vi "chaim Tx poulse.vi"() -> ()   [LabVIEW 2021]
doc: "This template is for the Simple NI-USRP Streaming design, a design that shows the basics of streaming data to and from an NI USRP-294x/295x device. Refer to the block diagram for more information about how to use this template."
uses:
  <vilib>/userDefined/Silver/nirio_resource_slv.ctl
  Host/SubVIs/Start Trigger.ctl
  <vilib>/Utility/error.llb/Error Cluster From Error Code.vi
  <vilib>/rvi/errors/niLvFpgaAdjustHostInterfaceError.vi
  <vilib>/rvi/interface/nirviReadWriteControl/nirviReadWriteControl.xnode
  <vilib>/rvi/interface/nirviMethod/nirviMethod.xnode
  NiFpgaLv.dll
  <vilib>/rvi/interface/Simulation/niFpgaSimulationCallBeginRW.vi
  <vilib>/FPGAPlugInAG/Dynamic/niLvFpga_WriteFifo_Dynamic.vi
  <vilib>/rvi/errors/niLvFpgaMergeErrorWithErrorCode.vi
panel:
  out "error out":errorcluster
  in  "stop":bool
  out "polse gen 1 params":T1
  out "pulse read polse gen 1":u32
  out "tx ocupaied":bool[](array[boolean])
  out "poulse param":T1
  out "pulse read":u32
  out "fpga clock":u64
  out "reset system clock":bool
  out "data":u64[](array[numeric]) format="%#.4e"
  out "Empty Elements Remaining":u32
  in  "file path":path
  in  "config tab":enum32{"Tx Configuration"}(tab)
  in  "tx config":T3={"rf enable 0"=TRUE, "rf config 0"={"antenna"="TX1", "frequency"=2000000000.0, "lo frequency"=-1.0, "level"=0.0}, "rf enable 1"=TRUE, "rf config 1"={"antenna"="TX1", "frequency"=2000000000.0, "lo frequency"=-1.0, "level"=0.0}, "transfer mode"=enum."Finite", "sample rate"=10000000.0, "number of samples"=8192, "start trigger"=enum."Immediate", "tone frequency"=100000.0} {"tone frequency" format="%#.3pHz"; "sample rate" format="%#.3pS/s"; "rf config 0"."level" format="%#_gdBm"; "rf config 0"."lo frequency" format="%#.3pHz"; "rf config 0"."frequency" format="%#.3pHz"; "rf config 1"."level" format="%#_gdBm"; "rf config 1"."lo frequency" format="%#.3pHz"; "rf config 1"."frequency" format="%#.3pHz"}
  in  "USRP RIO device":T4="RIO0" caption="USRP RIO Device"
  in  "reference frequency source":string(combo)="Internal" caption="Reference Frequency Source"
  in  "indicator tab":T5(tab)
  out "tx.output waveform":waveform(dbl)[](graph) caption="Output Waveform"
  out "tx.coerced config":T6 caption="Tx" {"coerced sample rates" format="%#.3pS/s"; "coerced levels" format="%#.3gdBm"; "coerced lo frequencies" format="%#.3pHz"; "coerced frequencies" format="%#.3pHz"}
  # "This template is for the Simple NI-USRP Streaming design, a design that shows the basics of streaming data on a USRP RIO device. See the block diagram for more information on how to use this template."
  # "Simple Tx Streaming"
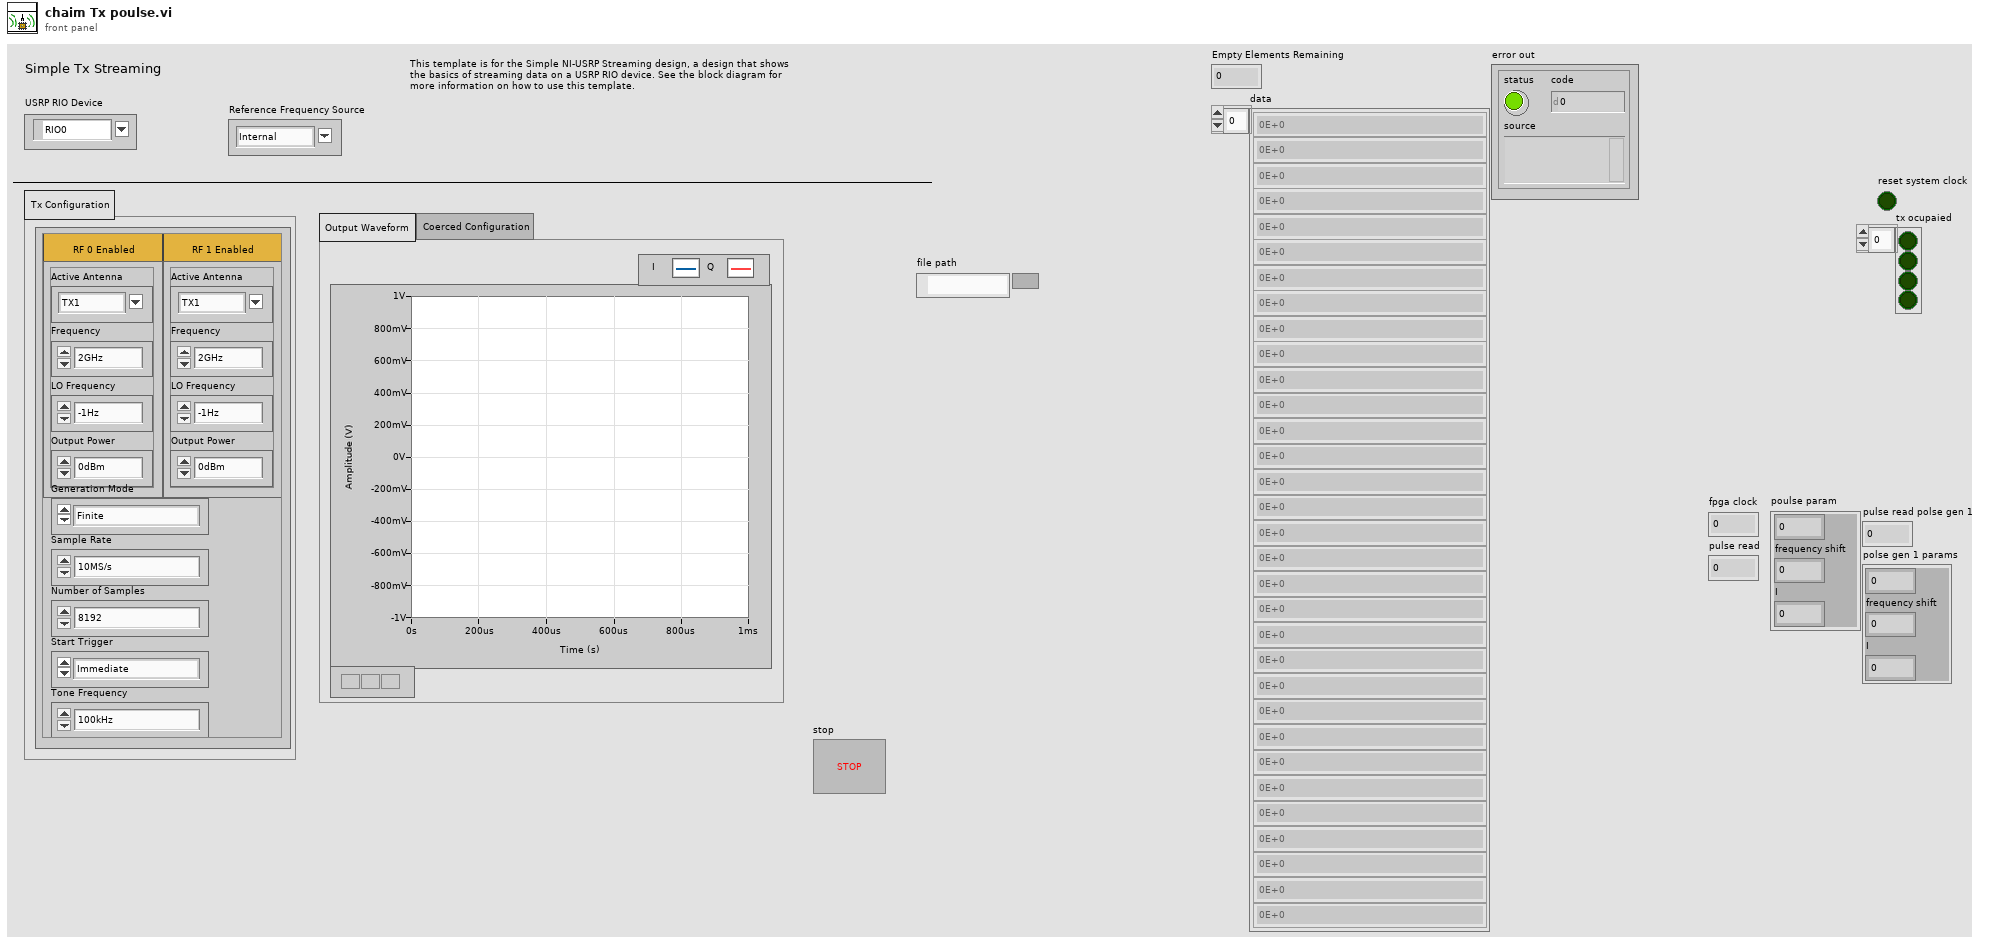
[diagram p1: front panel]
types:
  T1 = cluster{u32, "frequency shift":fxp<+/-,48,0>, "I":fxp<+/-,18,1>}
  T2 = typedef "Start Trigger.ctl" = enum8{"Software", "Digital Edge", "Rx Start Trigger", "Tx Start Trigger", "Immediate", "Future Time Event"}
  T3 = cluster{"rf enable 0":bool, "rf config 0":cluster{"antenna":string, "frequency":dbl, "lo frequency":dbl, "level":dbl}, "rf enable 1":bool, "rf config 1":cluster{"antenna":string, "frequency":dbl, "lo frequency":dbl, "level":dbl}, "transfer mode":enum16{"Finite", "Continuous"}, "sample rate":dbl, "number of samples":u32, "start trigger":T2, "tone frequency":dbl}
  T4 = typedef "nirio_resource_slv.ctl" = tag
  T5 = enum32{"Output Waveform", "Coerced Configuration"}
  T6 = cluster{"coerced frequencies":dbl[], "coerced lo frequencies":dbl[], "coerced levels":dbl[], "coerced sample rates":dbl[]}
  T7 = typedef "Tx Channels.ctl" = cluster{"tx config":cluster{"channel configuration":cluster{"channel enable":bool, "channel configuration":cluster{"antenna":string, "frequency":dbl, "lo frequency":dbl, "level":dbl}}[], "transfer mode":enum16{"Finite", "Continuous"}, "sample rate":dbl, "number of samples":u32, "start trigger":T2, "tone frequency":dbl}, "reference frequency source":string, "tx.data source":enum16{"SFP Port 0", "SFP Port 1", "Host"}, "tx.enabled channels":string[], "I":i16[], "Q":i16[], "tx.coerced configurations":cluster{"coerced frequencies":dbl[], "coerced lo frequencies":dbl[], "coerced levels":dbl[], "coerced sample rates":dbl[]}}
  T8 = typedef "niUsrpRio Config v1 Host.lvlib/niUsrpRio Session.ctl" = cluster{"FPGA Interface":refnum<k20>, "RIO Interface Number":u32, "Data Clock Rate":u32, "FPGA Data Clock Rate":u32, "Global Settings Register Bus":T9, "Radio 0 Settings Register Bus":T9, "Radio 1 Settings Register Bus":T9, "Radio Settings Bus Semaphore":T10, "DB Queues":T11[], "Characterization Data Valid?":bool, "EEPROM Header":T12, "Device Data Header":T13, "EEPROM Characterization Header":T14, "Characterization Data":T15[], "FPGA Current Version":u32, "FPGA Oldest Compatible Version":u32, "Fixed Logic Current Version":u32, "Fixed Logic Oldest Compatible Version":u32, "FPGA Radio Settings Bus Current Version":u32, "FPGA Radio Settings Bus Oldest Compatible Version":u32, "FPGA Board Config Current Version":u32, "FPGA Board Config Oldest Compatible Version":u32, "Daughterboard Clock Rate":u32, "daughterboard configuration session handles":u64[]}
  T9 = typedef "niInstr Register Bus v0 Host.lvlib/Register Bus Session.ctl" = refnum<queue>
  T10 = typedef "Semaphore RefNum" = refnum<k1>
  T11 = typedef "niUsrpRio Config v1 Host.lvlib/DB Queue Reference.ctl" = refnum<queue>
  T12 = typedef "niUsrpRio Config v1 Host.lvlib/EEPROM Header.ctl" = cluster{"Checksum":u32, "Product Code":u16, "Hardware Current Version":u16, "Hardware Oldest Compatible Version":u16, "EEPROM Map Current Version":u16, "EEPROM Map Oldest Compatible Version":u16, "User Password":string, "Pointer to Factory Header":u32, "Pointer to User Header":u32, "Recommended Interval":u16, "Number of Reserved Bytes":i32, "Number of Daughterboards":u8, "Daughterboard IDs":u16[], "Daughterboard Serial Numbers":string[]}
  T13 = typedef "niUsrpRio Config v1 Host.lvlib/EEPROM Device Data Header.ctl" = cluster{"Checksum":u32, "Number of Channels":u8, "Number of Gain Settings":u16[], "Pointer to Characterization Data":u32[], "Number of Reserved Bytes":i32, "Number of Frequencies":u16[]}
  T14 = typedef "niUsrpRio Config v1 Host.lvlib/EEPROM Characterization Header.ctl" = cluster{"Checksum":u32, "Date":timestamp, "Temperature":sgl, "Misc. Info":string, "Pointer to Device Data Header":u32, "Number of Reserved Bytes":i32}
  T15 = typedef "niUsrpRio Config v1 Host.lvlib/Characterization Data.ctl" = cluster{"Gains[dB]":dbl[], "Frequencies [Hz]":dbl[], "IQ Imbalance Table":T16[], "Measured Gains[dB]":dbl[][]}
  T16 = typedef "niUsrpRio Config v1 Host.lvlib/IQ Imbalance.ctl" = cluster{"Gain Imbalance [linear]":dbl, "Phase Imbalance [radians]":dbl, "Offset":cdb}
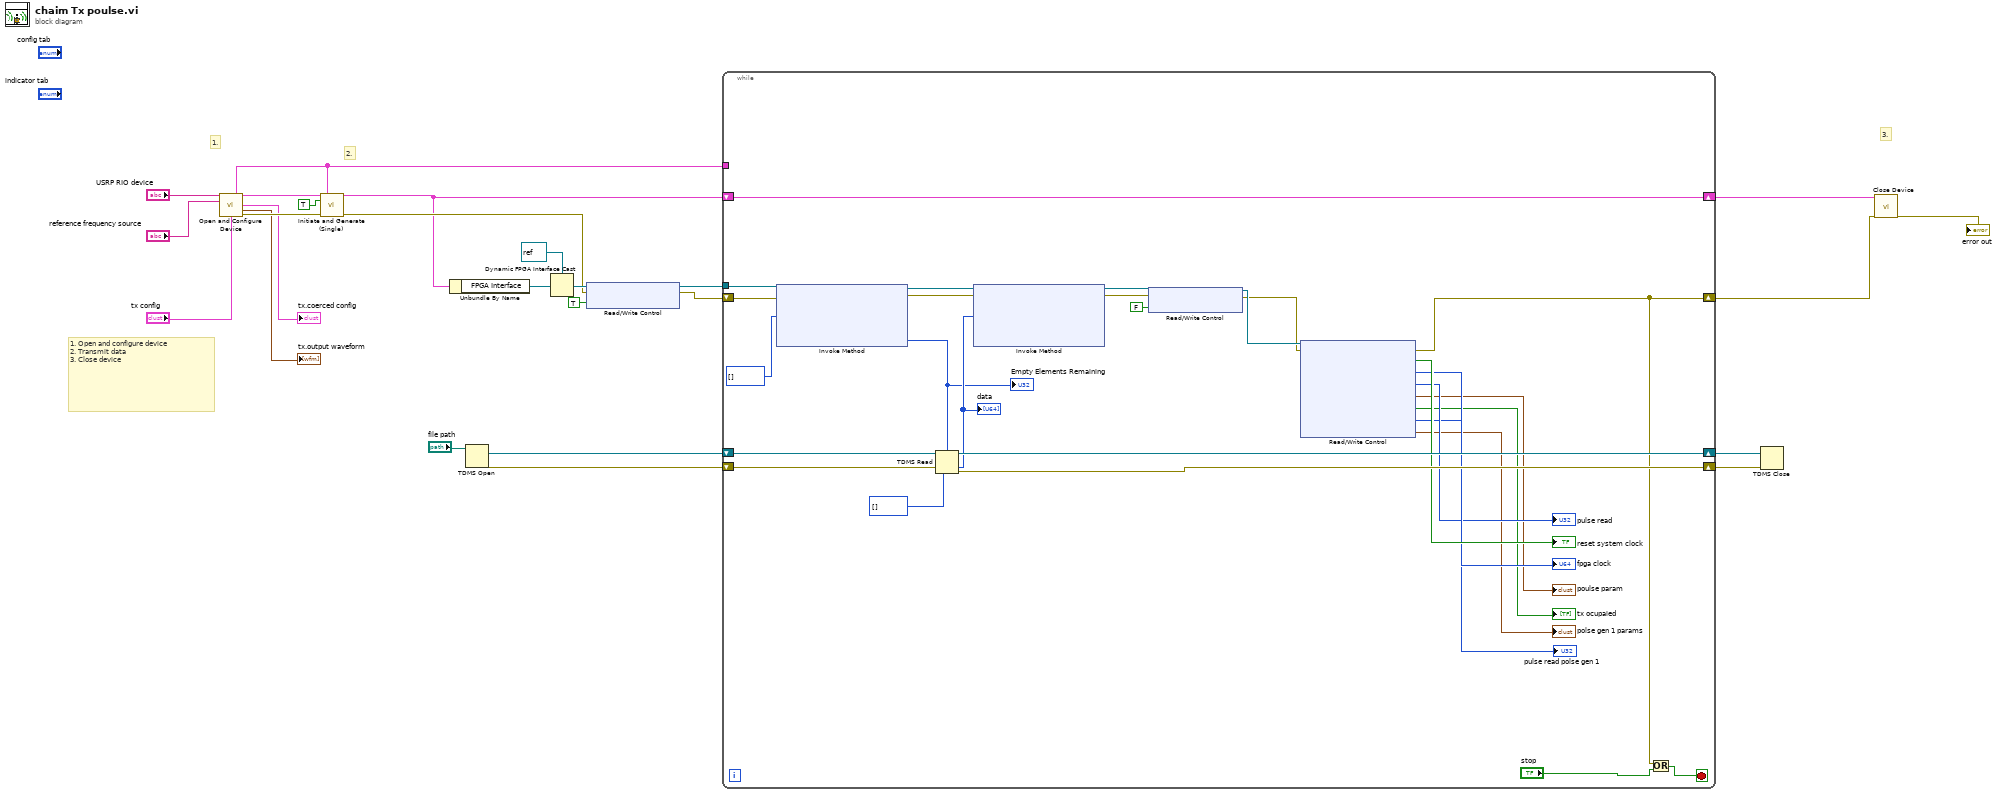
[diagram p0: block diagram]
diagram:
  # "2."
  # "3."
  # "1. Open and configure device\n2. Transmit data\n3. Close device"
  # "1."
  n1 = call "Open and Configure Device.vi"("USRP RIO Device"="USRP RIO device", "reference frequency source"="reference frequency source", "tx config"="tx config") -> ("tx channels"=w1:T7, "niUsrpRio Session (out)"=w18:T8, "tx.coerced configurations"=→"tx.coerced config":T6, "tx.output waveform"=→"tx.output waveform":waveform(dbl)[], "error out"=w25:errorcluster)  [unwired: 6 in, 2 out]
  n2 = call "Initiate and Generate (Single).vi"("niUsrpRio Session"=w18, "tx channels"=w1, "first iteration"=TRUE, "error in"=w25) -> ("niUsrpRio Session (out)"=w4:T8, "error out"=w7:errorcluster)  [unwired: 10 in]
  n3 = Unbundle By Name(w4) -> ("FPGA Interface"=w15:refnum<k20>)
  n4 = TDMS Open(11:"file path") -> (0:w11:errorcluster, 3:w12:refnum<k34>)  [unwired: 6 in]
  n5 = Dynamic FPGA Interface Cast(Session In=refnum<k20> refnum ("Type"), Type=w15) -> (Session Out=w14:refnum<k20>)
  n6 = xnode "Read/Write Control"("FPGA VI Reference In"=w14, "error in"=w7, "reset system clock"=TRUE) -> ("FPGA VI Reference Out"=w6:refnum<k20>, "error out"=w5:errorcluster)
  n7 = while {
    tunnel: w6 -> [w44]
    tunnel: w1 -> [_]
    shift-right: [w47] -> w10
    shift-left: w12 -> [w49]
    shift-right: [w46] -> w9
    shift-left: w11 -> [w48]
    shift-right: [w28] -> w2
    shift-left: w5 -> [w43]
    shift-right: [w37] -> w3
    shift-left: w4 -> [w37]
    stop <- w26 stop-if-true
    n8 = xnode "Invoke Method"("FPGA VI Reference In"=w44, "error in"=w43, "Data"=u64[] []) -> ("FPGA VI Reference Out"=w42:refnum<k20>, "error out"=w41:errorcluster, "Empty Elements Remaining"=w40:u32)  [unwired: 1 in]
    "Empty Elements Remaining" <- w40
    n9 = TDMS Read(0:w49, 2:w40, 11:w48, 12:u64[] [] ("Data")) -> (4:w47:refnum<k34>, 10:w45:u64[], 15:w46:errorcluster)  [unwired: 4 in, 3 out]
    "data" <- w45
    n10 = xnode "Invoke Method"("FPGA VI Reference In"=w42, "error in"=w41, "Data"=w45) -> ("FPGA VI Reference Out"=w51:refnum<k20>, "error out"=w52:errorcluster)  [unwired: 1 in, 1 out]
    n11 = xnode "Read/Write Control"("FPGA VI Reference In"=w51, "error in"=w52, "reset system clock"=FALSE) -> ("FPGA VI Reference Out"=w38:refnum<k20>, "error out"=w36:errorcluster)
    n12 = xnode "Read/Write Control"("FPGA VI Reference In"=w38, "error in"=w36) -> ("error out"=w28:errorcluster, "reset system clock"=→"reset system clock":bool, "fpga clock"=→"fpga clock":u64, "pulse read"=→"pulse read":u32, "poulse param"=→"poulse param":T1, "tx ocupaied"=→"tx ocupaied":bool[], "pulse read polse gen 1"=→"pulse read polse gen 1":u32, "polse gen 1 params"=→"polse gen 1 params":T1)  [unwired: 1 out]
    n13 = Or(x=w28, y="stop") -> (x .or. y?=w26:bool)
  }
  n14 = TDMS Close(8:w9, 11:w10) -> ()  [unwired: 2 out]
  n15 = call "Close Device.vi"("niUsrpRio Session"=w3, "error in"=w2) -> ("error out"=→"error out":errorcluster)  [unwired: 13 in]
